vi "Parse RW.vi"(8 "error in (no error)":errorcluster, 11 "R/W mode in":string) -> (0 "error out":errorcluster, 3 "R/W?":T1)   [LabVIEW 2018, in "File Parser Interface.lvlib" / "File Parser Interface.lvclass"]
uses:
  File Parser Interface.lvclass
  Ctls/RW Options.ctl
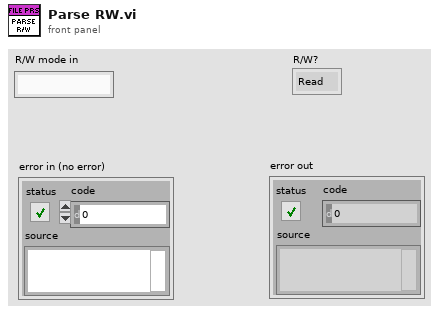
[diagram p1: front panel]
types:
  T1 = typedef "RW Options.ctl" = enum16{"Read", "Write", "R/W"}
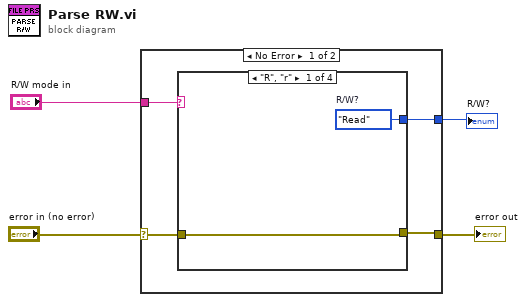
[diagram p0: block diagram]
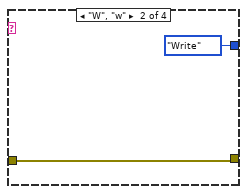
[diagram p2: hidden frame]
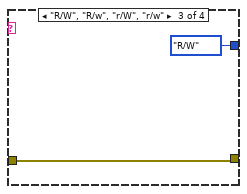
[diagram p3: hidden frame]
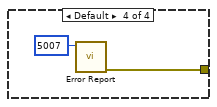
[diagram p4: hidden frame]
diagram:
  n1 = case shown="No Error" "error in (no error)" {
    selector: "error in (no error)" -> [w8 w17]
    tunnel: "R/W mode in" -> [w7 _]
    tunnel: [w6 w17] -> w2
    tunnel: [w5 _] -> w1
    frame No Error {
      n2 = case shown="\"R\", \"r\"" w7 {
        tunnel: w8 -> [w10 w12 w14 _]
        tunnel: [w10 w12 w14 w16] -> w6
        tunnel: [w9 RW_Options."Write" ("R/W?") RW_Options."R/W" ("R/W?") _] -> w5
        frame "R", "r" {
          w9 = RW_Options."Read"  # R/W?
        }
        frame "W", "w" {
        }
        frame "R/W", "R/w", "r/W", "r/w" {
        }
        frame Default {
          n3 = call "Error Report.vi"("Error Code"=i16 5007) -> ("error out"=w16:errorcluster)  [unwired: 10 in]
        }
      }
    }
    frame Error {
    }
  }
  "error out" <- w2
  "R/W?" <- w1
